vi "MQTT Receive message.vi"(7 "Topics":string[](array[string]), 8 "Topic":string, 9 "PUBLISH in":refnum<class "PUBLISH.lvclass">, 10 "Accessors:Module ID":i32, 11 "Client in":refnum<class "Client.lvclass">) -> (0 "error out":errorcluster, 3 "Client out":refnum<class "Client.lvclass">)   [LabVIEW 2020, in "MQTT_Client.lvlib"]
uses:
  MQTT_Client.lvlib
  <vilib>/LabVIEW Open Source Project/MQTT Client/Client class/Client.lvclass
  C:/Program Files (x86)/National Instruments/LabVIEW 2020/vi.lib/LabVIEW Open Source Project/MQTT Connection/MQTT_Base/Base Class/MQTT_Base.lvclass
  <vilib>/LabVIEW Open Source Project/MQTT Control Packets/Control Packets/PUBLISH/PUBLISH.lvclass
  <vilib>/LabVIEW Open Source Project/MQTT Connection/MQTT_Base/Base Class/MQTT_Base.lvclass/MQTT_Base.ctl
  8ba02f12-0147-4eb7-831c-a1a026d55034.vi
  <vilib>/Comparison/Equal/Equal Functor/Equal Functor.lvclass
  <vilib>/LabVIEW Open Source Project/OpenSerializer/Serializer/Serializer.lvclass
  <vilib>/LabVIEW Open Source Project/MQTT Connection/MQTT_Base/Base Class/MQTT_Base.lvclass
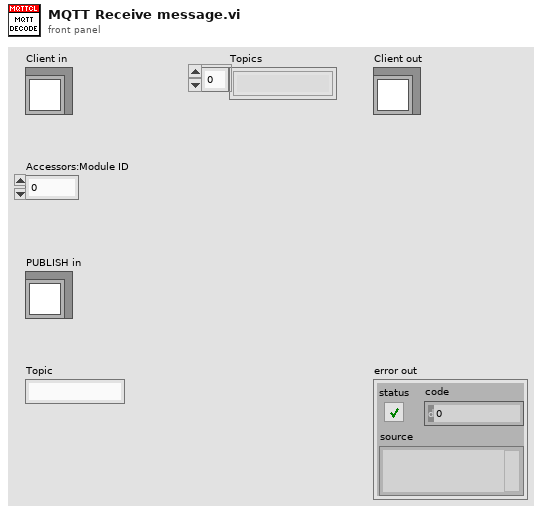
[diagram p1: front panel]
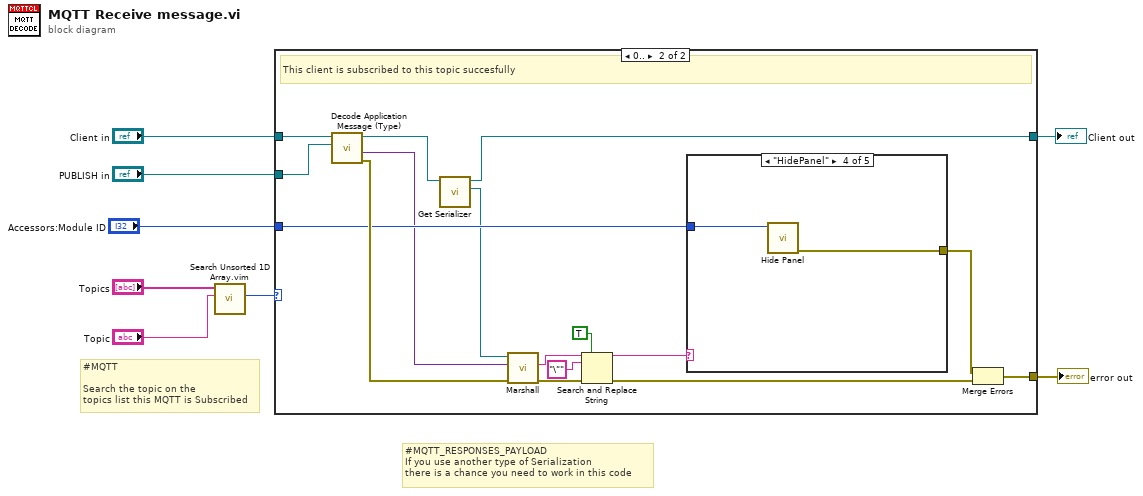
[diagram p0: block diagram]
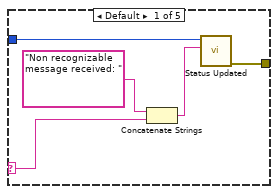
[diagram p3: hidden frame]
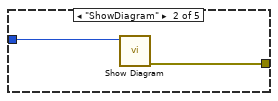
[diagram p4: hidden frame]
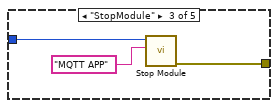
[diagram p5: hidden frame]
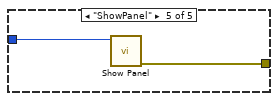
[diagram p6: hidden frame]
diagram:
  # "#MQTT_RESPONSES_PAYLOAD\nIf you use another type of Serialization\nthere is a chance you need to work in this code"
  # "#MQTT   \n\nSearch the topic on the \ntopics list this MQTT is Subscribed"
  n1 = call "Search Unsorted 1D Array.vim"("element"="Topic", "unsorted 1D array"="Topics") -> ("index of element"=w3:i32)  [unwired: 9 in]
  n2 = case shown="0.." w3 {
    tunnel: "Client in" -> [w9 w20]
    tunnel: "PUBLISH in" -> [_ w19]
    tunnel: [w9 w15] -> w6
    tunnel: [_ w25] -> w8
    tunnel: "Accessors:Module ID" -> [_ w18]
    frame ..-1 {
      # "Topic not found maybe need to subscribe"
    }
    frame 0.. {
      # "This client is subscribed to this topic succesfully"
      n3 = call <vilib>:"Decode Application Message (Type).vi"("PUBLISH"=w19, "Client in"=w20) -> ("error out"=w23:errorcluster, "Payload"=w17:variant, "Client out"=w16:refnum<class "Client.lvclass">)  [unwired: 6 in, 1 out]
      n4 = call <vilib>:"Get Serializer.vi"("MQTT_Base"=w16) -> ("Serializer"=w14:refnum<class "Serializer.lvclass">, "MQTT_Base out"=w15:refnum<class "Client.lvclass">)  [unwired: 8 in, 1 out]
      n5 = call <vilib>:"Marshall.vi"("error in (no error)"=w23, "Variant"=w17, "Serializer in"=w14) -> ("error out"=w22:errorcluster, "String"=w13:string)  [unwired: 6 in, 1 out]
      n6 = Search and Replace String(replace all?=TRUE ("replace all? (F)"), input string=w13, search string="\"", error in=w22) -> (result string=w10:string, error out=w21:errorcluster)  [unwired: 4 in, 2 out]
      n7 = case shown="\"HidePanel\"" w10 {
        selector: w10 -> [w30 _ _ _ _]
        tunnel: w18 -> [w28 w31 w34 w37 w38]
        tunnel: [w26 w32 w35 w36 w39] -> w24
        frame Default {
          n8 = Concatenate Strings("Non recognizable message received: " ("string"), w30) -> (w27:string)
          n9 = call "Status Updated.vi"("Status"=w27, "Module ID"=w28) -> ("error out"=w26:errorcluster)  [unwired: 9 in]
        }
        frame "ShowDiagram" {
          n10 = call "Show Diagram.vi"("Module ID"=w31) -> ("error out"=w32:errorcluster)  [unwired: 10 in]
        }
        frame "StopModule" {
          n11 = call "Stop Module.vi"("Origin"="MQTT APP", "Module ID"=w34) -> ("error out"=w35:errorcluster)  [unwired: 9 in]
        }
        frame "HidePanel" {
          n12 = call "Hide Panel.vi"("Module ID"=w37) -> ("error out"=w36:errorcluster)  [unwired: 10 in]
        }
        frame "ShowPanel" {
          n13 = call "Show Panel.vi"("Module ID"=w38) -> ("error out"=w39:errorcluster)  [unwired: 10 in]
        }
      }
      n14 = Merge Errors(w24, w21) -> (w25:errorcluster)
    }
  }
  "error out" <- w8
  "Client out" <- w6
